vi "Test Generated Voltage Ramp Length Correct.vi"(8 "error in (no error)":errorcluster, 11 "Ramp Voltage Test In":refnum<class "Ramp Voltage Test.lvclass">) -> (0 "error out":errorcluster, 3 "Ramp Voltage Test Out":refnum<class "Ramp Voltage Test.lvclass">)   [LabVIEW 2020, in "High Level PSU With Tests.lvlib" / "Ramp Voltage Test.lvclass"]
uses:
  Ramp Voltage Test.lvclass
  C:/Program Files (x86)/National Instruments/LabVIEW 2020/vi.lib/Astemes/LUnit/Test Case.lvclass
  Ramp Voltage/Ramp Settings.ctl
  <vilib>/Astemes/LUnit/Test Case.lvclass/Test Case.ctl
  01074fa8-ee8a-411d-bc8b-fc92c4f90959.vi
  <vilib>/Astemes/LUnit/Palette/Pass.vi
  <vilib>/Astemes/LUnit/Palette/Fail.vi
  <vilib>/Astemes/LUnit/Compare Variants.vi
  <vilib>/Astemes/LUnit/Describe Comparison.vi
  <vilib>/Astemes/LUnit/Set Assertion Type.vi
  <vilib>/Astemes/LUnit/Add test result.vi
  <vilib>/Astemes/LUnit/Variant to string.vi
  <vilib>/Astemes/LUnit/LUnit Record Assertion Result.vi
  <vilib>/Astemes/LUnit/LUnit Aggregate Assertion Results.vi
  <vilib>/Astemes/LUnit/Method Result/LUnit Merge Status.vi
  <vilib>/Astemes/LUnit/LUnit Concatenate result strings.vi
  <vilib>/Utility/Data Type/Get Type Information.vi
  <vilib>/Utility/LVClass/Get LV Class Name.vi
  Ramp Voltage Test.lvclass/Ramp Voltage Test.ctl
  Ramp Voltage/Ramp Voltage.lvclass
  Mock Voltage Output/Mock Voltage Output.lvclass
  C:/Git/astemes-gdevcon-2022/PSU Demo/High Level PSU With Tests/Mock Voltage Output/Mock Voltage Output.lvclass
  C:/Git/astemes-gdevcon-2022/PSU Demo/High Level PSU With Tests/Voltage Output/Voltage Output.lvclass
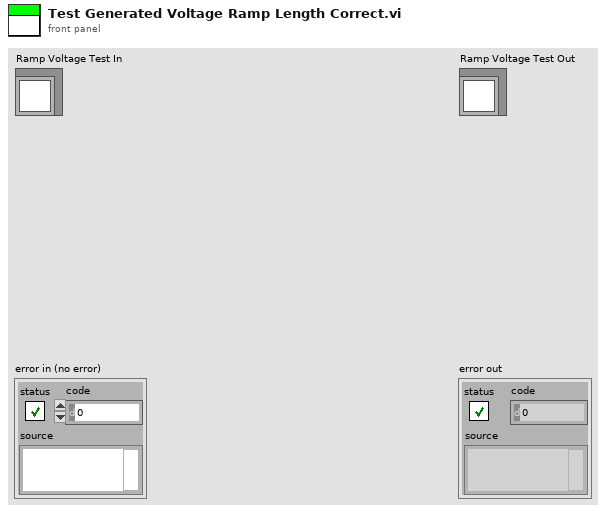
[diagram p1: front panel]
types:
  T1 = typedef "High Level PSU With Tests.lvlib/Ramp Voltage.lvclass/Ramp Settings.ctl" = cluster{"Max Output Voltage [V]":dbl, "Min Output Voltage [V]":dbl, "Step Size [V]":dbl, "Ramp Time [s]":dbl}
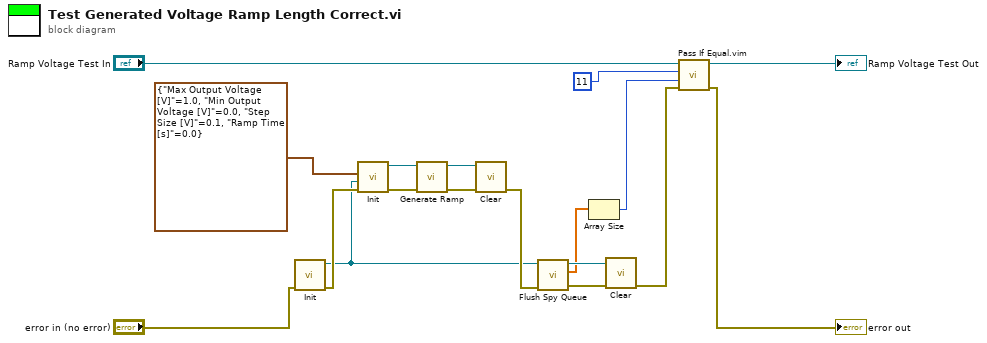
[diagram p0: block diagram]
diagram:
  n1 = call "Init.vi"("error in (no error)"="error in (no error)") -> ("error out"=w15:errorcluster, "Mock Voltage Output Out"=w5:refnum<class "Mock Voltage Output.lvclass">)  [unwired: 9 in]
  n2 = call "Init.vi"("error in (no error)"=w15, "Voltage Output"=w5, "Settings"=T1 {"Max Output Voltage [V]"=1.0, "Min Output Voltage [V]"=0.0, "Step Size [V]"=0.1, "Ramp Time [s]"=0.0}) -> ("error out"=w14:errorcluster, "Ramp Voltage Out"=w3:refnum<class "Ramp Voltage.lvclass">)  [unwired: 7 in]
  n3 = call "Generate Ramp.vi"("error in (no error)"=w14, "Ramp Use Case In"=w3) -> ("error out"=w4:errorcluster, "Ramp Use Case Out"=w2:refnum<class "Ramp Voltage.lvclass">)  [unwired: 8 in]
  n4 = call "Clear.vi"("error in (no error)"=w4, "Ramp Use Case in"=w2) -> ("error out"=w10:errorcluster)  [unwired: 8 in, 1 out]
  n5 = call "Flush Spy Queue.vi"("error in (no error)"=w10, "Mock Voltage Output in"=w5) -> ("error out"=w11:errorcluster, "Setpoints"=w8:dbl[], "Mock Voltage Output out"=w9:refnum<class "Mock Voltage Output.lvclass">)  [unwired: 7 in]
  n6 = Array Size(array=w8) -> (size(s)=w7:i32)
  n7 = call "Clear.vi"("error in (no error)"=w11, "Mock Voltage Output In"=w9) -> ("error out"=w12:errorcluster)  [unwired: 8 in, 1 out]
  n8 = call "Pass If Equal.vim"("error in (no error)"=w12, "Actual"=w7, "Expected"=11 ("size(s)"), "LUnit Test Case In"="Ramp Voltage Test In") -> ("error out"=→"error out":errorcluster, "LUnit Test Case Out"=→"Ramp Voltage Test Out":refnum<class "Ramp Voltage Test.lvclass">)  [unwired: 6 in]
